vi "OpenLabJackUtil (depreciated).vi"(6 "FirstFound":bool=TRUE, 7 "Address":string="192.168.1.209", 8 "error in":errorcluster, 9 "ConnectionType":u16(ring) items=["LJ_ctUSB", "LJ_ctETHERNET"], 10 "DeviceType":u16(ring)=1 items=["LJ_dtU3", "LJ_dtUE9"]) -> (0 "error out":errorcluster, 3 "Handle":i32)   [LabVIEW 2021]
panel:
  out "warning out":errorcluster
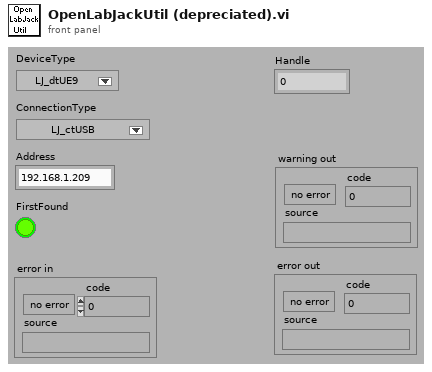
[diagram p1: front panel]
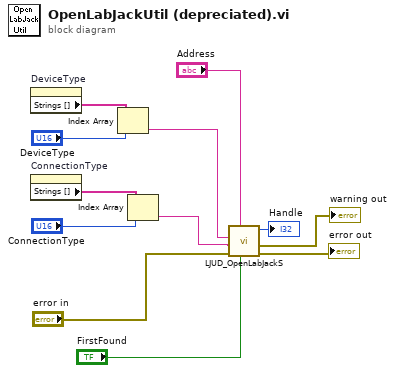
[diagram p0: block diagram]
diagram:
  n1 = property on="DeviceType" class="Ring (strict)"() -> ("Strings []"=w9:string[])  [unwired: 2 in, 2 out]
  n2 = property on="ConnectionType" class="Ring (strict)"() -> ("Strings []"=w7:string[])  [unwired: 2 in, 2 out]
  n3 = Index Array(array=w9, index="DeviceType") -> (element=w3:string)
  n4 = Index Array(array=w7, index="ConnectionType") -> (element=w2:string)
  n5 = call "LJUD_OpenLabJackS.vi"("FirstFound"="FirstFound", "Address"="Address", "error in"="error in", "ConnectionType"=w2, "DeviceType"=w3) -> ("error out"=→"error out":errorcluster, "warning out"=→"warning out":errorcluster, "Handle"=→"Handle":i32)  [unwired: 4 in]
